vi "get_samples_to_read.vi"(8 "error in (no error)":errorcluster, 11 "GenericSignalReader in":refnum<class "GenericSignalReader.lvclass">) -> (0 "error out":errorcluster, 1 "samples read":i32, 2 "total samples to read":i32, 3 "GenericSignalReader out":refnum<class "GenericSignalReader.lvclass">, 4 "samples still to be read":i32)   [LabVIEW 2010, in "GenericSignalReader.lvclass"]
uses:
  GenericSignalReader.lvclass
  GenericSignalReader.lvclass/GenericSignalReader.ctl
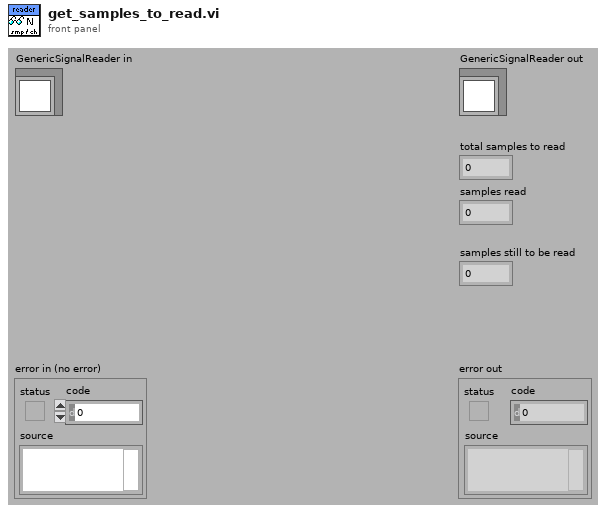
[diagram p1: front panel]
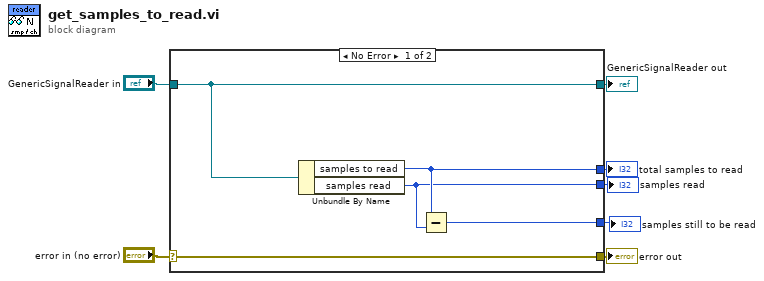
[diagram p0: block diagram]
diagram:
  n1 = case shown="No Error" "error in (no error)" {
    selector: "error in (no error)" -> [w12 w13]
    tunnel: [w12 w13] -> w6
    tunnel: [w11 w14] -> w4
    tunnel: "GenericSignalReader in" -> [w11 w14]
    tunnel: [w10 _] -> w3
    tunnel: [w9 _] -> w2
    tunnel: [w8 _] -> w1
    frame No Error {
      n2 = Unbundle By Name(w11) -> ("samples to read"=w10:i32, "samples read"=w9:i32)
      n3 = Subtract(x=w10, y=w9) -> (x-y=w8:i32)
    }
    frame Error {
    }
  }
  "error out" <- w6
  "GenericSignalReader out" <- w4
  "total samples to read" <- w3
  "samples read" <- w2
  "samples still to be read" <- w1
